vi "Create_AO_Signal.vi"(8 "error in":errorcluster, 10 "AO (%)":dbl(slide) min=0.0 max=100.0 step=1.0 scale=0.0..100.0, 11 "ON / OFF":bool=TRUE) -> (0 "error out":errorcluster, 2 "Samples":u32, 3 "WF":u32[](array[numeric]))   [LabVIEW 2021]
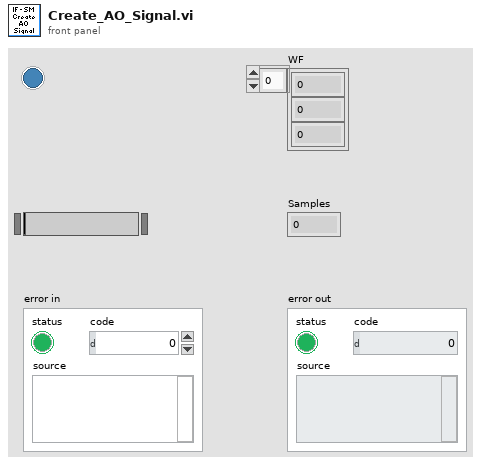
[diagram p1: front panel]
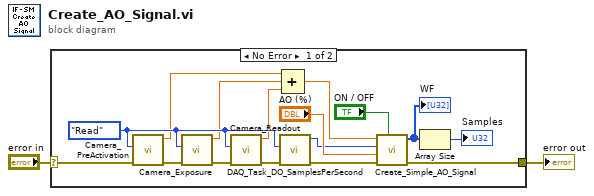
[diagram p0: block diagram]
diagram:
  n1 = case shown="No Error" "error in" {
    selector: "error in" -> [w17 w19]
    tunnel: [w5 w19] -> w1
    frame No Error {
      w14 = enum16{"Write", "Read"}."Read" ("Action")
      n2 = call "Camera_PreActivation.vi"("error in"=w17, "Action"=w14) -> ("error out"=w16:errorcluster, "Camera_PreActivation"=w10:dbl)  [unwired: 8 in]
      n3 = call "Camera_Exposure.vi"("error in"=w16, "Action"=w14) -> ("error out"=w15:errorcluster, "Exposure (s)"=w9:dbl)  [unwired: 8 in]
      n4 = call "Camera_Readout.vi"("error in"=w15, "Action"=w14) -> ("error out"=w13:errorcluster, "Camera_Readout"=w3:dbl)  [unwired: 8 in]
      n5 = call "DAQ_Task_DO_SamplesPerSecond.vi"("error in"=w13, "Action"=w14) -> ("error out"=w12:errorcluster, "DO_Task_SamplesPerSec"=w6:u32)  [unwired: 8 in]
      n6 = Compound Arithmetic op=ADD(w10, w9, w3) -> (w8:dbl)
      n7 = call "Create_Simple_AO_Signal.vi"("On/OFF"="ON / OFF", "error in"=w12, "Amplitude"="AO (%)", "Samples / s (10000)"=w6, "Time (s)"=w8) -> ("error out"=w5:errorcluster, "Signal"=w4:u32[])  [unwired: 5 in]
      "WF" <- w4
      n8 = Array Size(array=w4) -> (size(s)=→"Samples":i32)
    }
    frame Error {
    }
  }
  "error out" <- w1
